vi "FilterAirmarCompass.vi"(9 "Queue timeout (ms)":i32=200, 10 "NotifierReff":T1, 11 "AirmarGPS-Compass Queue Cluster":T2) -> ()   [LabVIEW 2013]
doc: "Performs and filtering that we want (default is no filtering) and writes the data to the notifier. If no data is in the queue this VI times out after 'Queue timeout (ms)' has passed and nothing is written to the notifier.\n\nEric Schneider, March 2014"
uses:
  Data/TypeDefs/GPS-Compass Queue Cluster.ctl
  Data/TypeDefs/UTM Location.ctl
  Data/TypeDefs/Notifiers.ctl
  Data/TypeDefs/Sail Set Suggestions.ctl
  Data/TypeDefs/Rudder Set Suggestions.ctl
  Data/TypeDefs/OverrideInformation.ctl
  Data/TypeDefs/OverrideMode.ctl
  Data/TypeDefs/MotorSetup.ctl
  Data/TypeDefs/DynamixelSetupInfo.ctl
  Data/TypeDefs/AirmarStatus.ctl
  Data/TypeDefs/HardwareOnline.ctl
  Data/TypeDefs/DynamixelCycleTracker.ctl
  Data/TypeDefs/RC Input Values.ctl
  Classes/Waypoint/Waypoint.lvclass
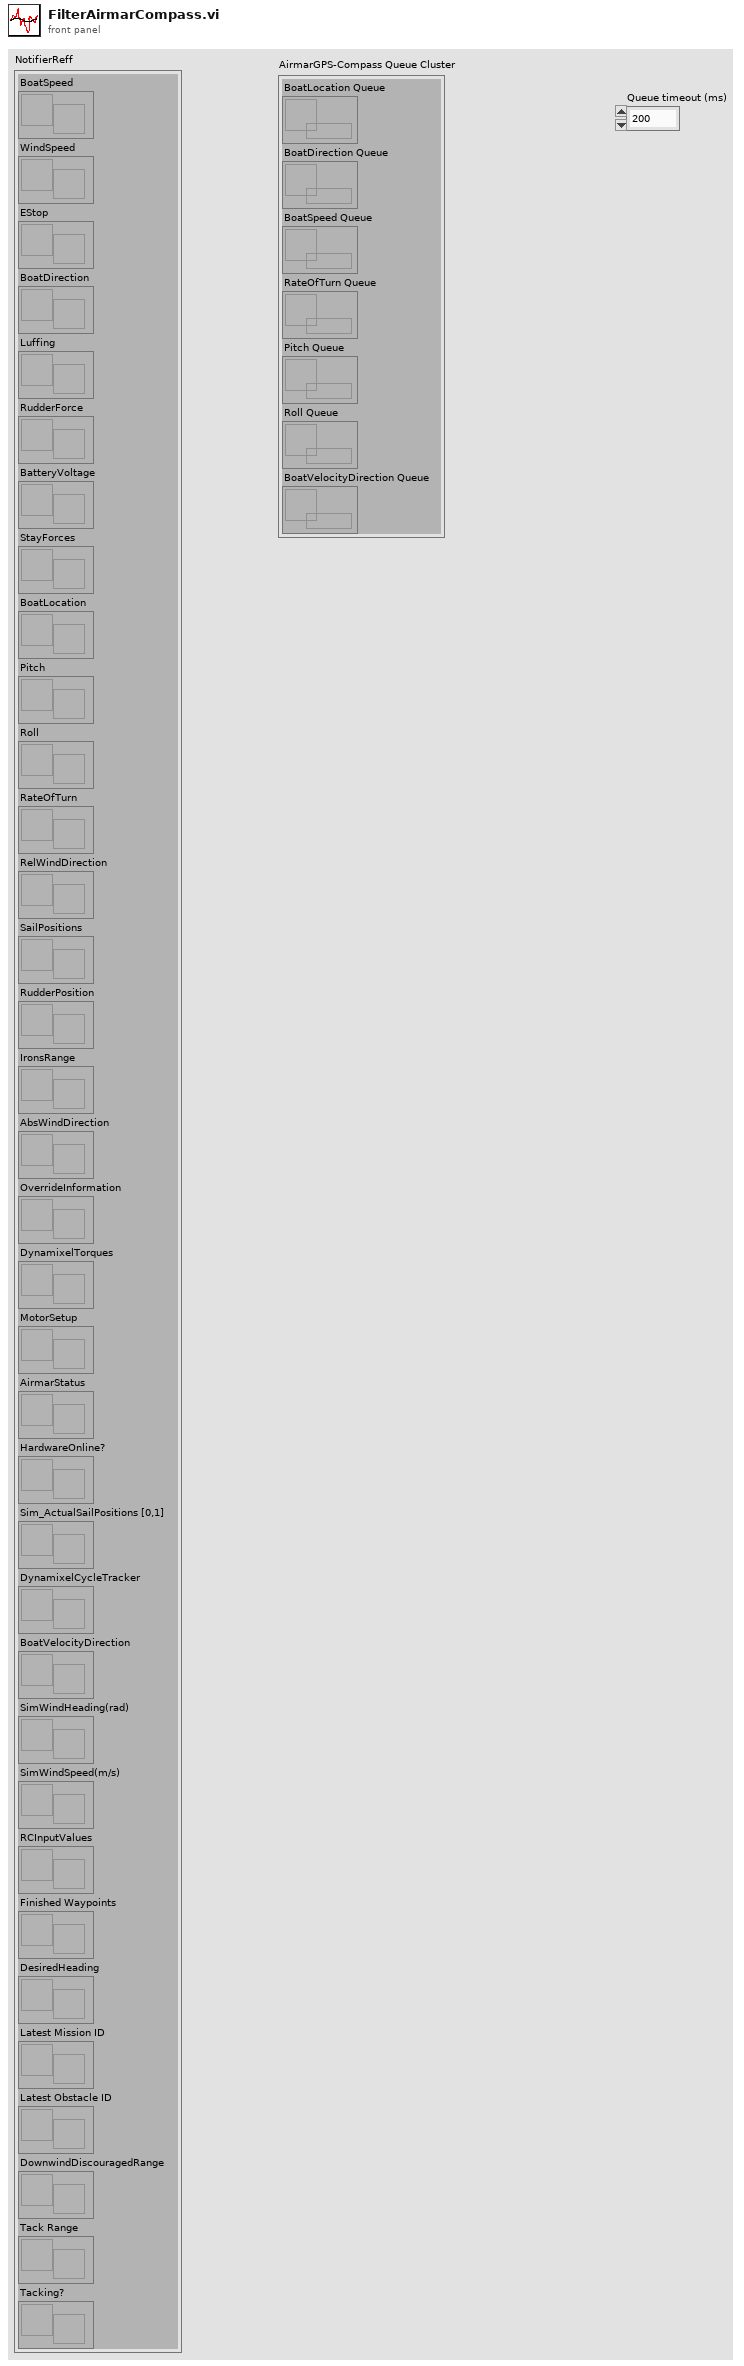
[diagram p1: front panel]
types:
  T1 = typedef "Notifiers.ctl" = cluster{"BoatSpeed":refnum<notifier>, "WindSpeed":refnum<notifier>, "EStop":refnum<notifier>, "BoatDirection":refnum<notifier>, "Luffing":refnum<notifier>, "RudderForce":refnum<notifier>, "BatteryVoltage":refnum<notifier>, "StayForces":refnum<notifier>, "BoatLocation":refnum<notifier>, "Pitch":refnum<notifier>, "Roll":refnum<notifier>, "RateOfTurn":refnum<notifier>, "RelWindDirection":refnum<notifier>, "SailPositions":refnum<notifier>, "RudderPosition":refnum<notifier>, "IronsRange":refnum<notifier>, "AbsWindDirection":refnum<notifier>, "OverrideInformation":refnum<notifier>, "DynamixelTorques":refnum<notifier>, "MotorSetup":refnum<notifier>, "AirmarStatus":refnum<notifier>, "HardwareOnline?":refnum<notifier>, "Sim_ActualSailPositions [0,1]":refnum<notifier>, "DynamixelCycleTracker":refnum<notifier>, "BoatVelocityDirection":refnum<notifier>, "SimWindHeading(rad)":refnum<notifier>, "SimWindSpeed(m/s)":refnum<notifier>, "RCInputValues":refnum<notifier>, "Finished Waypoints":refnum<notifier>, "DesiredHeading":refnum<notifier>, "Latest Mission ID":refnum<notifier>, "Latest Obstacle ID":refnum<notifier>, "DownwindDiscouragedRange":refnum<notifier>, "Tack Range":refnum<notifier>, "Tacking?":refnum<notifier>}
  T2 = typedef "GPS-Compass Queue Cluster.ctl" = cluster{"BoatLocation Queue":refnum<queue>, "BoatDirection Queue":refnum<queue>, "BoatSpeed Queue":refnum<queue>, "RateOfTurn Queue":refnum<queue>, "Pitch Queue":refnum<queue>, "Roll Queue":refnum<queue>, "BoatVelocityDirection Queue ":refnum<queue>}
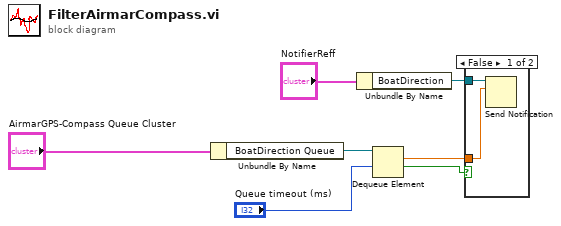
[diagram p0: block diagram]
diagram:
  n1 = Unbundle By Name("AirmarGPS-Compass Queue Cluster") -> ("BoatDirection Queue"=w6:refnum<queue>)
  n2 = Unbundle By Name("NotifierReff") -> ("BoatDirection"=w4:refnum<notifier>)
  n3 = Dequeue Element(queue=w6, timeout in ms (-1)="Queue timeout (ms)") -> (element=w1:dbl, timed out?=w2:bool)  [unwired: 1 in, 2 out]
  n4 = case shown="False" w2 {
    tunnel: w1 -> [w9 _]
    tunnel: w4 -> [w8 _]
    frame False {
      n5 = Send Notification(notification=w9, notifier=w8) -> ()  [unwired: 1 in, 2 out]
    }
    frame True {
    }
  }
